vi "Camera_Capture_Init.vi"(8 "Continuous?":T1, 9 "Detect Movement":bool, 10 "Crop?":bool, 11 "input cluster":T3={"L16 Linear Actuator"="", "XE 1000 Pump"="", "Camera1"="", "Camera2"="", "Camera1_IMG"=refnum, "Camera2_IMG"=refnum, "Img_Capt"=FALSE, "Actuator"=FALSE, "Pump"=FALSE, "Cam 1"=FALSE, "Cam 2"=FALSE, "Empty_Refill"=FALSE, "Crop"=FALSE, "Light intensity"=100, "Exposure Time"=1000.0, "Sample Name"="Test Sample", "Operator"="MRJ", "Calibration 1"=path "C:/Users/au540322/Desktop/IHS_Project/images/Debris/Debris_0/Debris_0_2019_06_01-23-32-49-686.PNG", "Calibration 2"=path "C:/Users/au540322/Desktop/IHS_Project/images/Debris/Debris_0/Debris_0_2019_06_01-23-32-49-686.PNG", "Framerate"=1, "Timeout Sample"=200, "Collection date"="", "Sample size threshold"=1, "Empty start"=1, "Command"="MRJ", "Calibration Image 1"=refnum, "Calibration Image 2"=refnum, "Original Image 1"=refnum, "Original Image 2"=refnum, "Processing Image 1"=refnum, "Processing Image 2"=refnum, "Object Image 1"=refnum, "Object Image 2"=refnum, "Cam 1 - save queue"=refnum, "Cam 2 - save queue"=refnum, "Station"="", "Species Name"="", "Other Notes"="", "Aperture"=enum."Item 0", "Image Process Queue Size"=500, "Image Save Queue Size"=500, "Overload threshold"=500, "Max Framerate"=100, "Blue Plane Image"=refnum, "Subtract Image"=refnum, "Binary Image 1"=refnum, "ROI mask allocation"=refnum, "Rectangle 1"={"Left"=0, "Top"=0, "Right"=0, "Bottom"=0, "Rotation"=0.0}, "Rectangle 2"={"Left"=0, "Top"=0, "Right"=0, "Bottom"=0, "Rotation"=0.0}, "Binary Image 2"=refnum, "Detection Region %"=0.0, "Cam 1 queue"=refnum, "Cam 2 queue"=refnum, "Detect image 1"=refnum, "Detect image 2"=refnum, "Detect 1"=path "C:/Users/au540322/Desktop/IHS_Project/images/Debris/Debris_0/Debris_0_2019_06_01-23-32-49-686.PNG", "Detect 2"=path "C:/Users/au540322/Desktop/IHS_Project/images/Debris/Debris_0/Debris_0_2019_06_01-23-32-49-686.PNG", "Max large object threshold"=0, "Open(T)/Close(F)"=FALSE} {"Rectangle 2"."Rotation" format="%.2f"; "Rectangle 2"."Left" scale=0.0..1024.0; "Rectangle 2"."Right" scale=0.0..1024.0; "Rectangle 1"."Rotation" format="%.2f"; "Rectangle 1"."Left" scale=0.0..1024.0; "Rectangle 1"."Right" scale=0.0..1024.0; "Max Framerate" min=1; "Overload threshold" min=1; "Image Save Queue Size" min=1; "Image Process Queue Size" min=1; "Empty start" min=1; "Sample size threshold" min=1; "Framerate" min=1; "Light intensity" scale=0.0..100.0}) -> (2 "Camera2":T2, 3 "Camera1":T2)   [LabVIEW 2019]
uses:
  controls/Data.ctl
  <vilib>/userdefined/High Color/IMAQdx.ctl
  <vilib>/vision/Image Controls.llb/IMAQ Image.ctl
  <vilib>/vision/driver/IMAQdx.llb/IMAQdx Acquisition Mode.ctl
  Camera_ID.ctl
  <vilib>/vision/driver/NI_Vision_Acquisition_Software.lvlib
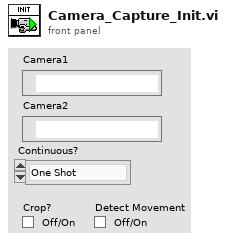
[diagram p1: front panel]
types:
  T1 = typedef "NI_Vision_Acquisition_Software.lvlib/IMAQdx Acquisition Mode.ctl" = enum32{"One Shot", "Continuous"}
  T2 = typedef "IMAQdx.ctl" = refnum<k21>
  T3 = typedef "Data.ctl" = cluster{"L16 Linear Actuator":refnum<visa-resource-name>, "XE 1000 Pump":refnum<visa-resource-name>, "Camera1":T2, "Camera2":T2, "Camera1_IMG":T4, "Camera2_IMG":T4, "Img_Capt":bool, "Actuator":bool, "Pump":bool, "Cam 1":bool, "Cam 2":bool, "Empty_Refill":bool, "Crop":bool, "Light intensity":i32, "Exposure Time":dbl, "Sample Name":string, "Operator":string, "Calibration 1":path, "Calibration 2":path, "Framerate":i32, "Timeout Sample":i32, "Collection date":string, "Sample size threshold":i32, "Empty start":u32, "Command":string, "Calibration Image 1":T4, "Calibration Image 2":T4, "Original Image 1":T4, "Original Image 2":T4, "Processing Image 1":T4, "Processing Image 2":T4, "Object Image 1":T4, "Object Image 2":T4, "Cam 1 - save queue":refnum<queue>, "Cam 2 - save queue":refnum<queue>, "Station":string, "Species Name":string, "Other Notes":string, "Aperture":enum32{"Item 0", "Item 1", "Item 2", "Item 3"}, "Image Process Queue Size":i32, "Image Save Queue Size":i32, "Overload threshold":i32, "Max Framerate":i32, "Blue Plane Image":T4, "Subtract Image":T4, "Binary Image 1":T4, "ROI mask allocation":T4, "Rectangle 1":T5, "Rectangle 2":T5, "Binary Image 2":T4, "Detection Region %":dbl, "Cam 1 queue":refnum<queue>, "Cam 2 queue":refnum<queue>, "Detect image 1":T4, "Detect image 2":T4, "Detect 1":path, "Detect 2":path, "Max large object threshold":i32, "Open(T)/Close(F)":bool}
  T4 = typedef "IMAQ Image.ctl" = refnum<image>
  T5 = typedef "IMAQ Rectangle" = cluster{"Left":i32, "Top":i32, "Right":i32, "Bottom":i32, "Rotation":dbl}
  T6 = typedef "Camera_ID.ctl" = enum16{"Camera 1", "Camera 2"}
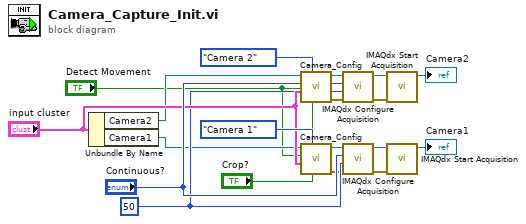
[diagram p0: block diagram]
diagram:
  w15 = u32 50 ("Number of Buffers")
  n1 = Unbundle By Name("input cluster") -> ("Camera2"=w4:T2, "Camera1"=w3:T2)
  n2 = call "Camera_Config.vi"("Crop?"="Crop?", "Camera"=Camera_ID."Camera 2", "input cluster"="input cluster", "Detect Movement"="Detect Movement", "Refnum in"=w4) -> ("error out"=w12:errorcluster, "Refnum out"=w14:T2)  [unwired: 4 in]
  n3 = call "Camera_Config.vi"("Crop?"="Crop?", "Camera"=Camera_ID."Camera 1", "input cluster"="input cluster", "Detect Movement"="Detect Movement", "Refnum in"=w3) -> ("error out"=w8:errorcluster, "Refnum out"=w9:T2)  [unwired: 4 in]
  n4 = call <vilib>:"IMAQdx Configure Acquisition.vi"("error in"=w12, "Number of Buffers"=w15, "Continuous?"="Continuous?", "Session In"=w14) -> ("error out"=w11:errorcluster, "Session Out"=w13:T2)  [unwired: 6 in]
  n5 = call <vilib>:"IMAQdx Configure Acquisition.vi"("error in"=w8, "Number of Buffers"=w15, "Continuous?"="Continuous?", "Session In"=w9) -> ("error out"=w6:errorcluster, "Session Out"=w7:T2)  [unwired: 6 in]
  n6 = call <vilib>:"IMAQdx Start Acquisition.vi"("error in"=w11, "Session In"=w13) -> ("Session Out"=→"Camera2":T2)  [unwired: 8 in, 1 out]
  n7 = call <vilib>:"IMAQdx Start Acquisition.vi"("error in"=w6, "Session In"=w7) -> ("Session Out"=→"Camera1":T2)  [unwired: 8 in, 1 out]
